vi "Add Routing Channel (Template) RTM.vi"(8 "error in (no error)":errorcluster, 11 "Node Ptr":u64 format="%.0x") -> (0 "error out":errorcluster)   [LabVIEW 2020, in "Routing and Faulting System Explorer.lvlib"]
uses:
  Routing and Faulting System Explorer.lvlib
  Scripting/Routing and Faulting Scripting.lvlib
  <vilib>/NI VeriStand/Custom Device Tools/Custom Device Utility Library/Custom Device Utility Library.lvlib
  <vilib>/NI VeriStand/Custom Device API/Custom Device API.lvlib
panel:
  in  "Tag":string
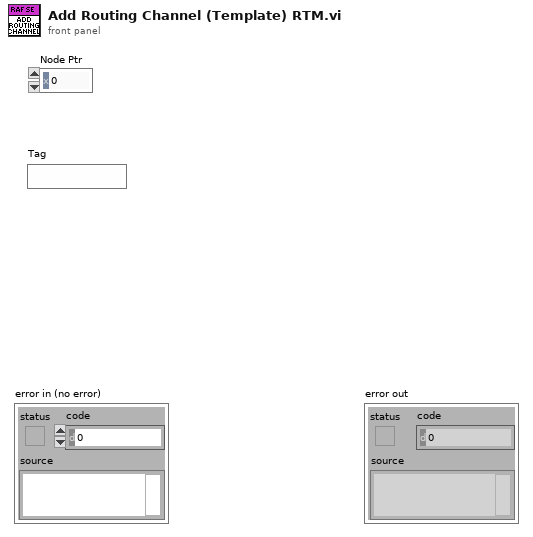
[diagram p1: front panel]
types:
  T1 = typedef "Custom Device API.lvlib/Custom Device Item Ref.ctl" = u64
  T2 = typedef "Routing and Faulting Scripting.lvlib/Module Information.ctl" = cluster{"Module Path":string, "Product Name":string, "Possible Connections":T3[], "Configuration Revision":u32, "Validated":bool, "Missing":bool}
  T3 = typedef "Routing and Faulting Hardware API.lvlib/Possible Connections for Endpoint.ctl" = cluster{"Source":string, "Destinations":string[]}
  T4 = typedef "Routing and Faulting Shared.lvlib/Channel States.ctl" = T5[]
  T5 = typedef "Routing and Faulting Shared.lvlib/Routing State.ctl" = cluster{"Name":string, "Description":string, "Value":i32, "Connection List":T6[]}
  T6 = typedef "Routing and Faulting Shared.lvlib/Connection.ctl" = cluster{"Module":string, "Source":string, "Destination":string}
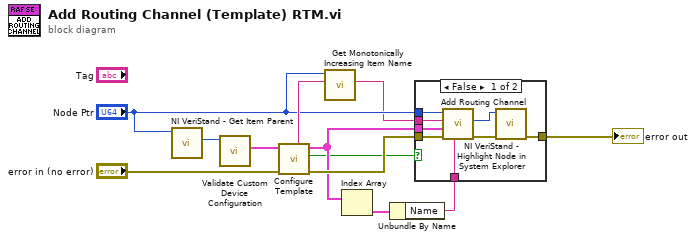
[diagram p0: block diagram]
diagram:
  n1 = call <vilib>:"NI VeriStand - Get Item Parent.vi"("Item Ref in"="Node Ptr") -> ("Parent Ref"=w11:T1)  [unwired: 7 in, 3 out]
  n2 = call "Validate Custom Device Configuration.vi"("Routing and Faulting Custom Device Ref"=w11) -> ("Module Connection Information"=w10:T2[])  [unwired: 8 in, 2 out]
  n3 = call "Configure Template.vi"("error in"="error in (no error)", "Module Connection Information"=w10) -> ("error out"=w9:errorcluster, "Cancelled?"=w5:bool, "State Configurations"=w7:T4, "Routing Channel Name"=w3:string)  [unwired: 6 in]
  n4 = call "Get Monotonically Increasing Item Name.vi"("Desired Name"=w3, "Section Ptr"="Node Ptr") -> ("New Item Name"=w1:string)  [unwired: 7 in, 2 out]
  n5 = Index Array(array=w7) -> (element=w6:T5)  [unwired: 1 in]
  n6 = Unbundle By Name(w6) -> ("Name"=w4:string)
  n7 = case shown="False" w5 {
    tunnel: "Node Ptr" -> [w20 _]
    tunnel: w1 -> [w19 _]
    tunnel: [w17 w21] -> w8
    tunnel: w7 -> [w15 _]
    tunnel: w9 -> [w14 w21]
    tunnel: w4 -> [w13 _]
    frame False {
      n8 = call "Add Routing Channel.vi"("initial state"=w13, "error in"=w14, "state configurations"=w15, "channel name"=w19, "routing channels in"=w20) -> ("error out"=w18:errorcluster, "routing channel"=w16:T1)  [unwired: 4 in, 1 out]
      n9 = call <vilib>:"NI VeriStand - Highlight Node in System Explorer.vi"("error in (no error)"=w18, "Item Ref in"=w16) -> ("error out"=w17:errorcluster)  [unwired: 8 in, 1 out]
    }
    frame True {
    }
  }
  "error out" <- w8
